vi "Finish Environment.vi"(8 "error in (no error)":errorcluster, 11 "Test Framework in":refnum<class "Test Framework.lvclass">) -> (0 "error out":errorcluster, 3 "Test Framework out":refnum<class "Test Framework.lvclass">)   [LabVIEW 2020, in "Test Framework.lvclass"]
uses:
  Test Framework.lvclass
  Test Framework.lvclass/Test Framework.ctl
  Instruments/Power Supply/Power Supply.lvclass
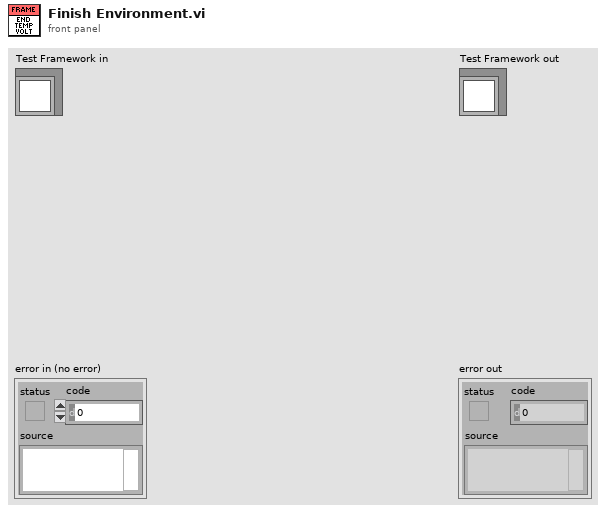
[diagram p1: front panel]
types:
  T1 = typedef "Test Framework.lvclass/Temperature and voltage array.ctl" = cluster{"Temperature [C]":dbl, "Soak time [m]":dbl, "PSUs":cluster{"Enabled":bool, "Source":enum32{"Voltage", "Current"}, "Drive (V/A)":dbl, "Sweep (V/A)":string, "Limit (A/V)":dbl, "PSU alias":string, "PSU info":cluster{"ID":string, "Address":string, "Channel":u8}}[]}[]
  T2 = typedef "Test Framework.lvclass/Temperature and voltage modes.ctl" = cluster{"Temperature mode":enum16{"Automatic", "Manual", "Off"}, "DC-Power mode":enum16{"Automatic", "Manual", "Off"}, "PSU sweep mode":bool, "Turn off after measurement":bool}
  T3 = cluster{"Temperature control array":T1, "Temperature mode":T2}
  T4 = cluster{"Temperature [C]":dbl, "Soak time [m]":dbl, "PSUs":cluster{"Enabled":bool, "Source":enum32{"Voltage", "Current"}, "Drive (V/A)":dbl, "Sweep (V/A)":string, "Limit (A/V)":dbl, "PSU alias":string, "PSU info":cluster{"ID":string, "Address":string, "Channel":u8}}[]}
  T5 = cluster{"Enabled":bool, "Source":enum32{"Voltage", "Current"}, "Drive (V/A)":dbl, "Sweep (V/A)":string, "Limit (A/V)":dbl, "PSU alias":string, "PSU info":cluster{"ID":string, "Address":string, "Channel":u8}}[]
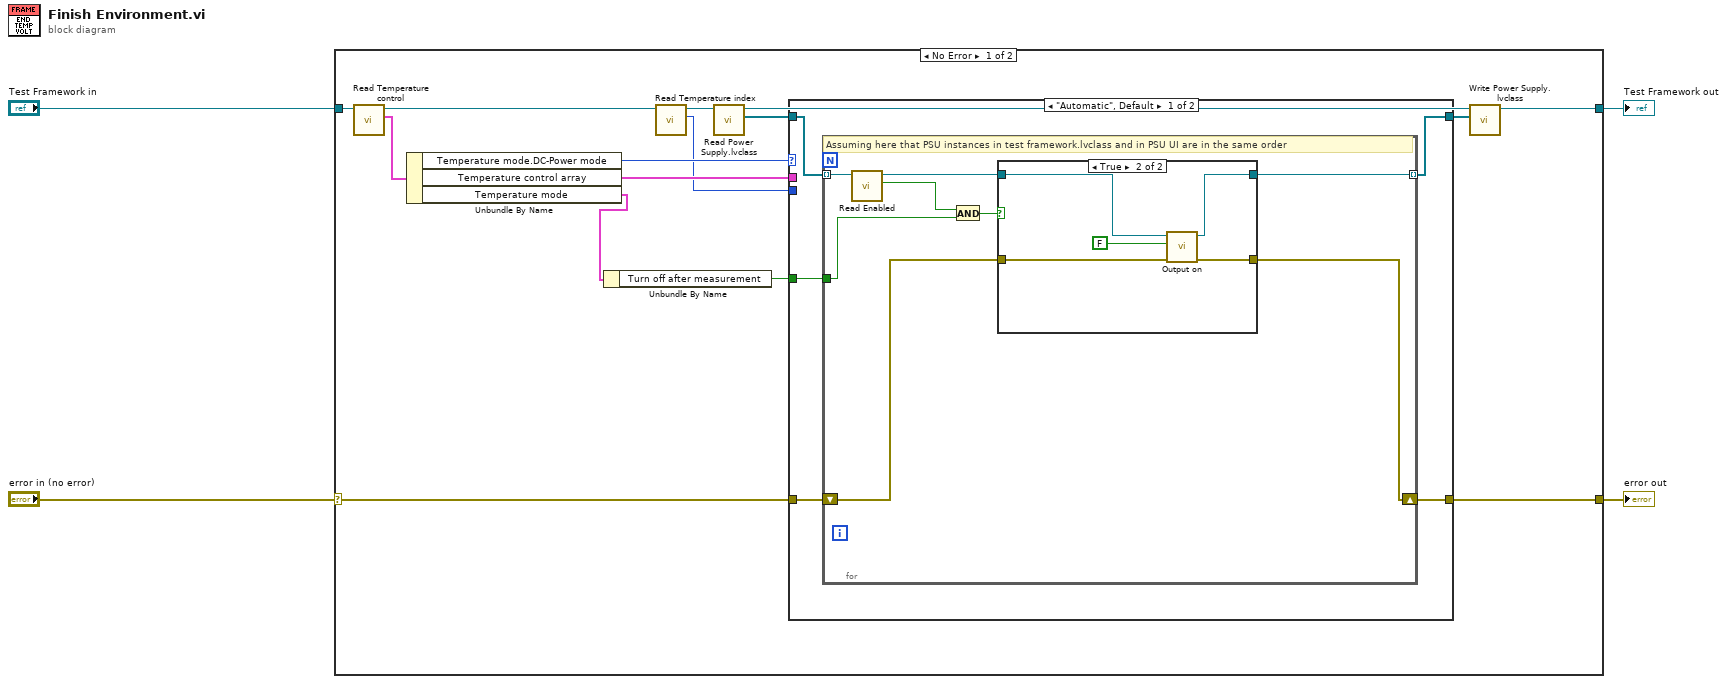
[diagram p0: block diagram]
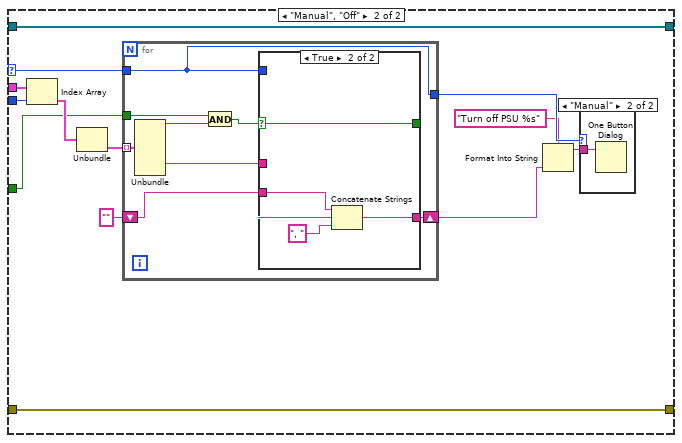
[diagram p3: hidden frame]
diagram:
  n1 = case shown="No Error" "error in (no error)" {
    selector: "error in (no error)" -> [w12 w69]
    tunnel: [w11 w69] -> w3
    tunnel: [w13 w68] -> w1
    tunnel: "Test Framework in" -> [w8 w68]
    frame No Error {
      n2 = call-dynamic "Read Temperature control.vi"("Test Framework in"=w8) -> ("Temperature control"=w19:T3, "Test Framework out"=w6:refnum<class "Test Framework.lvclass">)  [unwired: 9 in]
      n3 = Unbundle By Name(w19) -> ("Temperature mode.DC-Power mode"=w15:enum16{"Automatic", "Manual", "Off"}, "Temperature control array"=w9:T1, "Temperature mode"=w14:T2)
      n4 = Unbundle By Name(w14) -> ("Turn off after measurement"=w10:bool)
      n5 = call "Read Temperature index.vi"("Test Framework in"=w6) -> ("Environmental index"=w7:i32, "Test Framework out"=w5:refnum<class "Test Framework.lvclass">)  [unwired: 9 in]
      n6 = call "Read Power Supply.lvclass.vi"("Test Framework in"=w5) -> ("Power Supply lvclasses"=w16:refnum<class "Power Supply.lvclass">[], "Test Framework out"=w18:refnum<class "Test Framework.lvclass">)  [unwired: 9 in]
      n7 = case shown="\"Automatic\", Default" w15 {
        selector: w15 -> [_ w51]
        tunnel: w16 -> [w24 w50]
        tunnel: [w23 w52] -> w11
        tunnel: w12 -> [w22 w52]
        tunnel: [w21 w50] -> w17
        tunnel: w10 -> [w20 w41]
        tunnel: w9 -> [_ w49]
        tunnel: w7 -> [_ w40]
        frame "Automatic", Default {
          n8 = for {
            shift-right: [w31] -> w23
            shift-left: w22 -> [w30]
            tunnel: w24 -> [w29] mode=indexing
            tunnel: [w32] -> w21 mode=indexing
            tunnel: w20 -> [w27]
            # "Assuming here that PSU instances in test framework.lvclass and in PSU UI are in the same order"
            n9 = call-dynamic "Read Enabled.vi"("Power Supply in"=w29) -> ("Enabled"=w26:bool, "Power Supply out"=w28:refnum<class "Power Supply.lvclass">)  [unwired: 9 in]
            n10 = And(x=w26, y=w27) -> (x .and. y?=w25:bool)
            n11 = case shown="True" w25 {
              tunnel: w28 -> [w34 w37]
              tunnel: [w34 w39] -> w32
              tunnel: [w33 w38] -> w31
              tunnel: w30 -> [w33 w36]
              frame False {
                # "Disabled. Don't change anything."
              }
              frame True {
                n12 = call-dynamic "Output on.vi"("error in (no error)"=w36, "Output On"=FALSE, "Power Supply in"=w37) -> ("error out"=w38:errorcluster, "Power Supply out"=w39:refnum<class "Power Supply.lvclass">)  [unwired: 7 in]
              }
            }
          }
        }
        frame "Manual", "Off" {
          n13 = Index Array(array=w49, index=w40) -> (element=w48:T4)
          n14 = Unbundle(w48) -> ("PSUs"=w47:T5)  [unwired: 2 out]
          n15 = for {
            tunnel: w47 -> [w61] mode=indexing
            tunnel: w51 -> [w60]
            tunnel: [w60] -> w45
            shift-right: [w58] -> w43
            shift-left: "" -> [w57]
            tunnel: w41 -> [w56]
            n16 = Unbundle(w61) -> ("Enabled"=w55:bool, "PSU alias"=w59:string)  [unwired: 5 out]
            n17 = And(x=w56, y=w55) -> (x .and. y?=w54:bool)
            n18 = case shown="True" w54 {
              selector: w54 -> [_ w67]
              tunnel: w59 -> [_ w66]
              tunnel: [_ w67] -> _
              tunnel: w60 -> [_ _]
              tunnel: [w62 w64] -> w58
              tunnel: w57 -> [w62 w63]
              frame False {
              }
              frame True {
                n19 = Concatenate Strings(w63, w66, ", " ("string")) -> (w64:string)
              }
            }
          }
          n20 = Format Into String(format string="Turn off PSU %s", w43) -> (resulting string=w46:string)  [unwired: 2 in, 1 out]
          n21 = case shown="\"Manual\"" w45 {
            tunnel: w46 -> [_ w53]
            frame "Off", Default {
            }
            frame "Manual" {
              n22 = One Button Dialog(message=w53) -> ()  [unwired: 1 in, 1 out]
            }
          }
        }
      }
      n23 = call "Write Power Supply.lvclass.vi"("Power Supply lvclasses"=w17, "Test Framework in"=w18) -> ("Test Framework out"=w13:refnum<class "Test Framework.lvclass">)  [unwired: 9 in]
    }
    frame Error {
    }
  }
  "error out" <- w3
  "Test Framework out" <- w1
